vi "temp-global.vi"() -> ()   [LabVIEW 2013]
panel:
  in  "Temperature Array":dbl[](array[numeric])
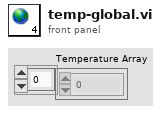
[diagram p1: front panel]
diagram:
